vi "Set_Parameter_Instrument (Json).vi"(8 "error in (no error)":errorcluster caption="entrée d'erreur (pas d'erreur)", 10 "Parameter (Json)":string, 11 "FW_Check_Hash_code en entrée":refnum<class "FW_Check_Hash_code.lvclass">) -> (0 "error out":errorcluster caption="sortie d'erreur", 3 "FW_Check_Hash_code en sortie":refnum<class "FW_Check_Hash_code.lvclass">)   [LabVIEW 2020, in "Library Test.lvlib" / "FW_Check_Hash_code.lvclass"]
uses:
  FW_Check_Hash_code.lvclass
  C:/Users/ngarcin/OneDrive - Altyor/Standard TB/Class/Test/Test (Default)/Test (Default).lvclass
  Commun VI/TypeDef/Commande Test/Commande Code Hash.ctl
  FW_Check_Hash_code.lvclass/FW_Check_Hash_code.ctl
  JSON API/JSON Value/Set from JSON string.vi
  Test_Without_Instr/Test_Without_Inst.lvclass
  JSON API/JSON Value/JSON Value.lvclass
  JSON API/Variant JSON/Variant JSON.lvlib
  JSON API/Get Polymorphic/JSON GetSet.lvlib
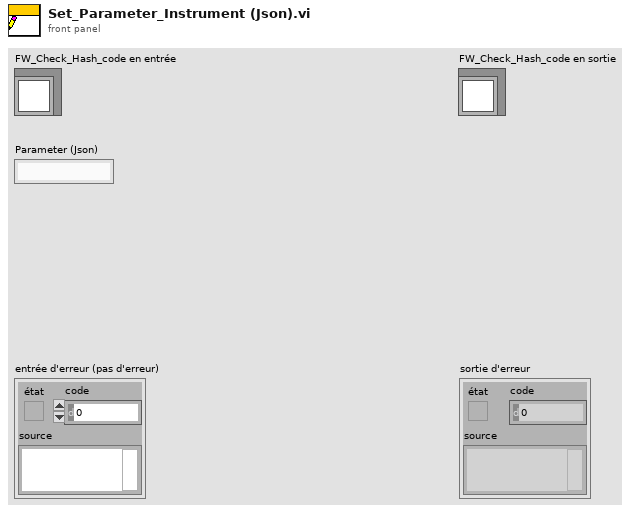
[diagram p1: front panel]
types:
  T1 = typedef "Commande Code Hash.ctl" = cluster{"Path FW ":path}
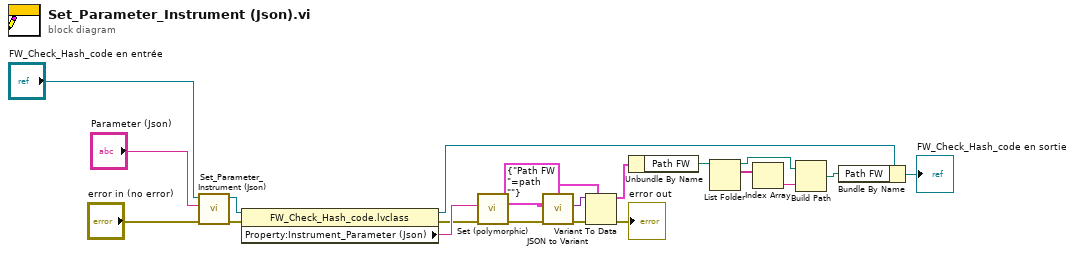
[diagram p0: block diagram]
diagram:
  w13 = T1 {"Path FW "=path ""}
  n1 = call-parent "Set_Parameter_Instrument (Json).vi"("error in (no error)"="error in (no error)", "Parameter (Json)"="Parameter (Json)", "Test (Default) en entrée"="FW_Check_Hash_code en entrée") -> ("error out"=w3:errorcluster, "Test (Default) en sortie"=w4:refnum<class "FW_Check_Hash_code.lvclass">)  [unwired: 7 in]
  n2 = property class="FW_Check_Hash_code.lvclass"(reference=w4, error in=w3) -> (reference out=w12:refnum<class "FW_Check_Hash_code.lvclass">, error out=w10:errorcluster, "Property:Instrument_Parameter (Json)"=w14:string)
  n3 = call-poly "Set (polymorphic).vi"("error in (no error)"=w10, "JSON stream"=w14) -> ("error out"=w16:errorcluster, "JSON Value out"=w18:refnum<class "JSON Value.lvclass">)  [unwired: 7 in, 1 out]
  n4 = call "JSON to Variant.vi"("error in (no error)"=w16, "Variant (Data Type)"=w13, "JSON Value"=w18) -> ("error out"=w17:errorcluster, "Variant out"=w15:variant)  [unwired: 7 in]
  n5 = Variant To Data(error in=w17, type=w13, Variant=w15) -> (data=w11:T1, error out=→"error out":errorcluster)
  n6 = Unbundle By Name(w11) -> ("Path FW"=w6:path)
  n7 = List Folder(path=w6) -> (path out=w7:path, filenames=w9:string[])  [unwired: 3 in, 2 out]
  n8 = Index Array(array=w9) -> (element=w8:string)  [unwired: 1 in]
  n9 = Build Path(base path=w7, name or relative path=w8) -> (appended path=w5:path)
  n10 = Bundle By Name(cluster=w12, "Path FW"=w5) -> (→"FW_Check_Hash_code en sortie":refnum<class "FW_Check_Hash_code.lvclass">)
